vi "Handle Notification.vi"(8 "error in (no error)":errorcluster, 9 "Payload":string, 10 "Notification Type":string, 11 "Waterfall in":refnum<class "Waterfall.lvclass">) -> (0 "error out":errorcluster, 3 "Waterfall out":refnum<class "Waterfall.lvclass">)   [LabVIEW 2024, in "Waterfall.lvlib" / "Waterfall.lvclass"]
uses:
  Waterfall.lvclass
  Waterfall.lvclass/Waterfall.ctl
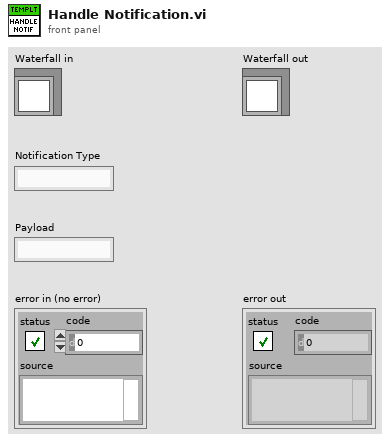
[diagram p1: front panel]
types:
  T1 = typedef "Waterfall.lvlib/Waterfall.lvclass/Waterfall Data.ctl" = cluster{"First Time":bool, "Show Waterfall Button Clicked":bool, "Data to Process":dbl, "Slice":dbl, "window":T2, "averaging parameters":cluster{"averaging mode":enum16{"No averaging", "Vector averaging", "RMS averaging", "Peak hold"}, "weighting mode":enum16{"Linear", "Exponential"}, "number of averages":u32}, "Waterfall VI Ref":refnum<vi>, "Signal":waveform(dbl)}
  T2 = typedef "NI_AALPro.lvlib/windowTd.ctl" = u32
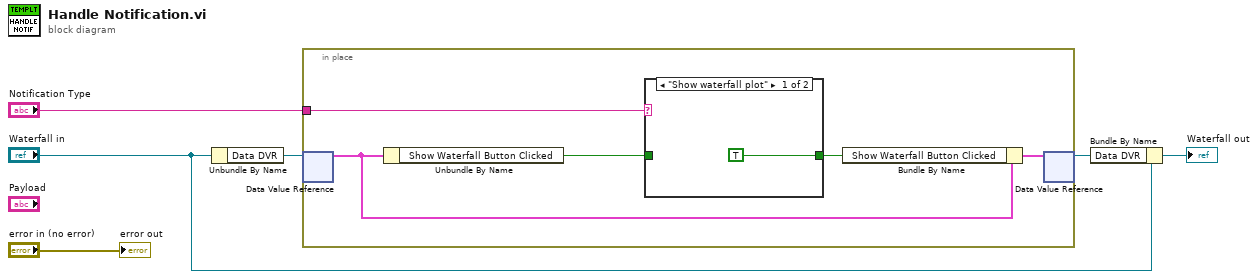
[diagram p0: block diagram]
diagram:
  n1 = Unbundle By Name("Waterfall in") -> ("Data DVR"=w6:refnum<data-value>)
  n2 = in-place {
    in-place-border: "Notification Type" -> [w11]
    n3 = in-place-dvr #1(w6) -> (w9:T1)  [unwired: 1 out]
    n4 = Unbundle By Name(w9) -> ("Show Waterfall Button Clicked"=w10:bool)
    n5 = case shown="\"Show waterfall plot\"" w11 {
      tunnel: w10 -> [_ w13]
      tunnel: [TRUE w13] -> w8
      frame "Show waterfall plot" {
      }
      frame Default {
      }
    }
    n6 = Bundle By Name(cluster=w9, "Show Waterfall Button Clicked"=w8) -> (w7:T1)
    n7 = in-place-dvr #1(w7) -> (w5:refnum<data-value>)  [unwired: 1 out]
  }
  n8 = Bundle By Name(cluster="Waterfall in", "Data DVR"=w5) -> (→"Waterfall out":refnum<class "Waterfall.lvclass">)
  "error out" <- "error in (no error)"
